vi "Ampint162Dbl.vi"(4 "In i16":u16) -> (1 "Amp (%)":dbl)   [LabVIEW 2013]
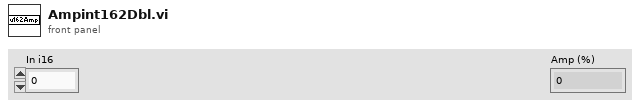
[diagram p1: front panel]
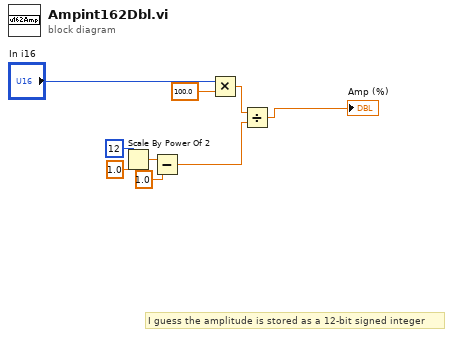
[diagram p0: block diagram]
diagram:
  # "I guess the amplitude is stored as a 12-bit signed integer"
  n1 = Scale By Power Of 2(n=i16 12, x=1.0) -> (x*2^n=w7:dbl)
  n2 = Subtract(x=w7, y=1.0) -> (x-y=w2:dbl)
  n3 = Multiply(x="In i16", y=100.0) -> (x*y=w3:dbl)
  n4 = Divide(x=w3, y=w2) -> (x/y=→"Amp (%)":dbl)
